vi "ARGBSetChannelValueCore.vi"(7 "Channel":T1, 8 "error in (no error)":errorcluster, 10 "Value":u8, 11 "Src":refnum<data-value>) -> (0 "error out":errorcluster)   [LabVIEW 2020, in "g_ar_toolkit.image.lvlib"]
uses:
  g_ar_toolkit.image.lvlib
  ARGBChannels.ctl
  bin/g_ar_toolkit.1.32.dll
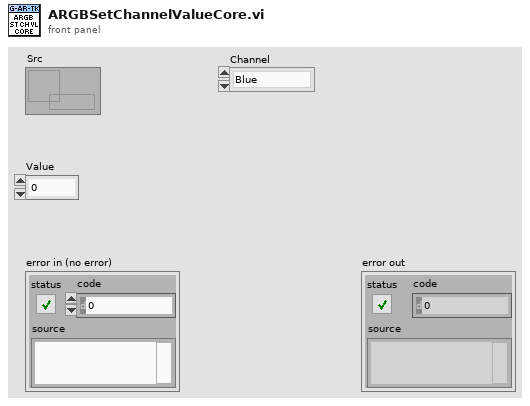
[diagram p1: front panel]
types:
  T1 = typedef "g_ar_toolkit.image.lvlib/ARGBChannels.ctl" = enum8{"Blue", "Green", "Red", "Alpha"}
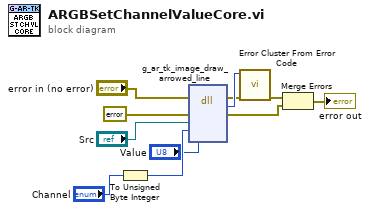
[diagram p0: block diagram]
diagram:
  n1 = To Unsigned Byte Integer(number="Channel") -> (unsigned 8bit integer=w2:u8)
  n2 = dll-call lib="C:/serenial/libraries/g-augmented-reality-toolkit/LabVIEW/bin/g_ar_toolkit.1.*.*" fn="g_ar_tk_image_draw_arrowed_line"(error in="error in (no error)", "error_cluster"=errorcluster {"status"=FALSE, "code"=0, "source"=""} ("error constant"), "EDVR src"="Src", "Channel"=w2, "Value"="Value") -> (error out=w4:errorcluster, "MgErr"=w5:i32, "error_cluster"=w8:errorcluster)  [unwired: 5 in, 1 out]
  n3 = call <vilib>:"Error Cluster From Error Code.vi"("error in (no error)"=w4, "error code (0)"=w5) -> ("error out"=w6:errorcluster)  [unwired: 7 in]
  n4 = Merge Errors(w6, w8) -> (→"error out":errorcluster)
